vi "Run Test.vi"(8 "error in (no error)":errorcluster, 10 "Test Run Request":refnum<class "Test Run Request.lvclass">, 11 "Generic Execution Adapter in":refnum<class "Generic Execution Adapter.lvclass">) -> (0 "error out":errorcluster, 2 "Test Run Result":refnum<class "Test Run Result.lvclass">, 3 "Generic Execution Adapter out":refnum<class "Generic Execution Adapter.lvclass">)   [LabVIEW 2026, in "Generic Execution Adapter.lvclass"]
uses:
  Generic Execution Adapter.lvclass
  Generic Execution Adapter.lvclass/Generic Execution Adapter.ctl
  c793dbd1-c522-441b-8e2b-9b0b2a24b1d8.vi
  Domain/Test Run Result/Test Run Result.lvclass
  Typedefs/enums/Run Outcome Enum.ctl
  Domain/Test Run Request/Test Run Request.lvclass
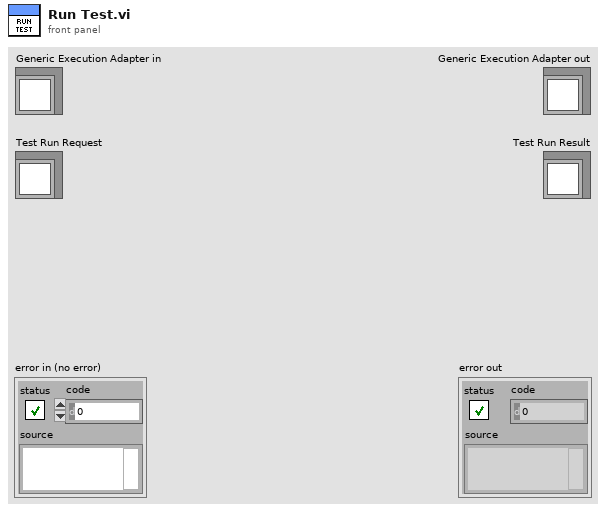
[diagram p1: front panel]
types:
  T1 = typedef "Run Outcome Enum.ctl" = enum16{"Unkown", "Passed", "Failed", "Error", "Aborted"}
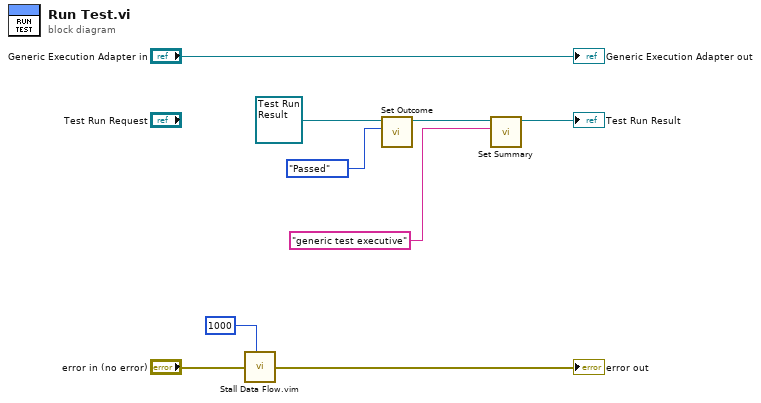
[diagram p0: block diagram]
diagram:
  n1 = call "Stall Data Flow.vim"("value in"="error in (no error)", "milliseconds to wait"=u32 1000) -> ("value out"=→"error out":errorcluster)  [unwired: 1 out]
  n2 = call "Set Outcome.vi"("Outcome"=Run_Outcome_Enum."Passed", "Test Run Result in"=refnum<class "Test Run Result.lvclass"> refnum) -> ("Test Run Result out"=w3:refnum<class "Test Run Result.lvclass">)  [unwired: 9 in]
  n3 = call "Set Summary.vi"("Summary"="generic test executive", "Test Run Result in"=w3) -> ("Test Run Result out"=→"Test Run Result":refnum<class "Test Run Result.lvclass">)  [unwired: 9 in]
  "Generic Execution Adapter out" <- "Generic Execution Adapter in"
